vi "x^2-8 sub.vi"(1 "x":dbl) -> (0 "sonuç":dbl)   [LabVIEW 2014]
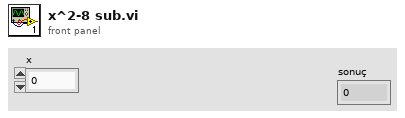
[diagram p1: front panel]
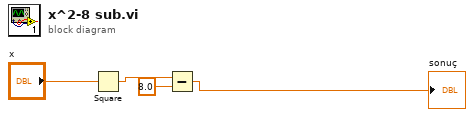
[diagram p0: block diagram]
diagram:
  n1 = Square(x="x") -> (x^2=w3:dbl)
  n2 = Subtract(x=w3, y=8.0) -> (x-y=→"sonuç":dbl)
